vi "Set Item TypeGUID.vi"(8 "error in (no error)":errorcluster, 10 "TypeGUID":string, 11 "Item Reference in":T1 format="%.0x") -> (0 "error out":errorcluster, 3 "Item Reference out":T1 format="%.0x")   [LabVIEW 2013, in "Hierarchy Framework.lvlib" / "Item.lvclass"]
uses:
  Item.lvclass
  Ctls/Item Reference.ctl
  Generic/Generic.lvclass
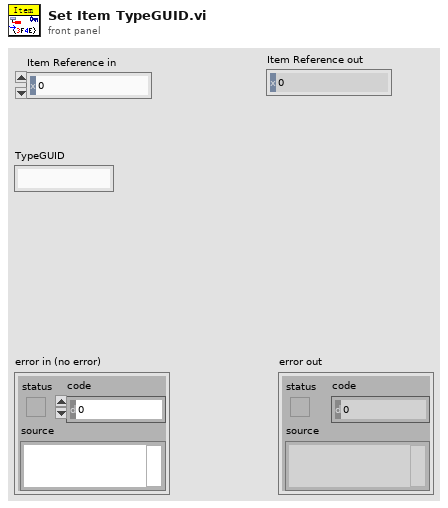
[diagram p1: front panel]
types:
  T1 = typedef "Hierarchy Framework.lvlib/Item.lvclass/Item Reference.ctl" = u64
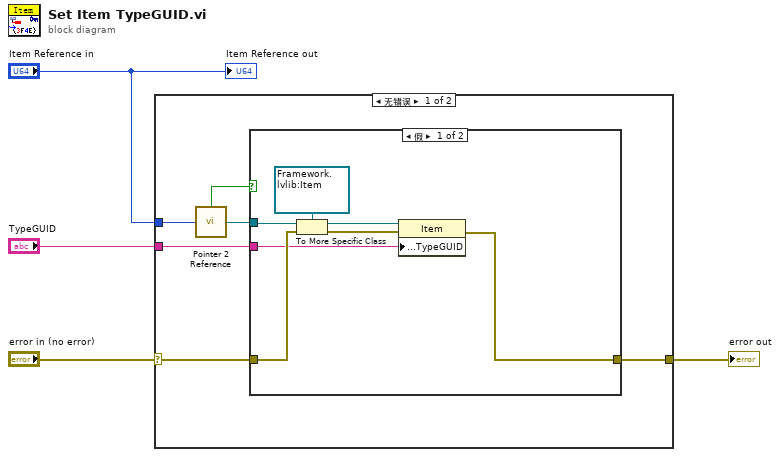
[diagram p0: block diagram]
diagram:
  n1 = case shown="无错误" "error in (no error)" {
    selector: "error in (no error)" -> [w9 w19]
    tunnel: "Item Reference in" -> [w8 _]
    tunnel: [w10 w19] -> w3
    tunnel: "TypeGUID" -> [w5 _]
    frame No Error {
      n2 = call "Pointer 2 Reference.vi"("Pointer"=w8) -> ("Not A Refnum?"=w7:bool, "Generic Reference"=w6:refnum<data-value>)
      n3 = case shown="假" w7 {
        tunnel: w9 -> [w16 w18]
        tunnel: [w12 w18] -> w10
        tunnel: w6 -> [w17 _]
        tunnel: w5 -> [w11 _]
        frame False {
          n4 = To More Specific Class(target class=refnum<data-value> refnum ("Item"), reference=w17, error in=w16) -> (specific class reference=w14:refnum<data-value>, error out=w13:errorcluster)
          n5 = property class="Item"(reference=w14, error in=w13, "Accessors:TypeGUID"=w11) -> (error out=w12:errorcluster)  [unwired: 1 out]
        }
        frame True {
        }
      }
    }
    frame Error {
    }
  }
  "error out" <- w3
  "Item Reference out" <- "Item Reference in"
